vi "Destroy.vi"(0 "reference in":refnum<class "GSwFormDSP.lvclass">, 5 "error in (no error)":errorcluster) -> (14 "reference out":refnum<class "GSwFormDSP.lvclass">, 19 "error out":errorcluster)   [LabVIEW 2022 SP3, in "GSwFormDSP.lvclass"]
doc: "Destructor."
uses:
  GSwFormDSP.lvclass
  Generic Utilities_class/Generic Utilities.lvclass
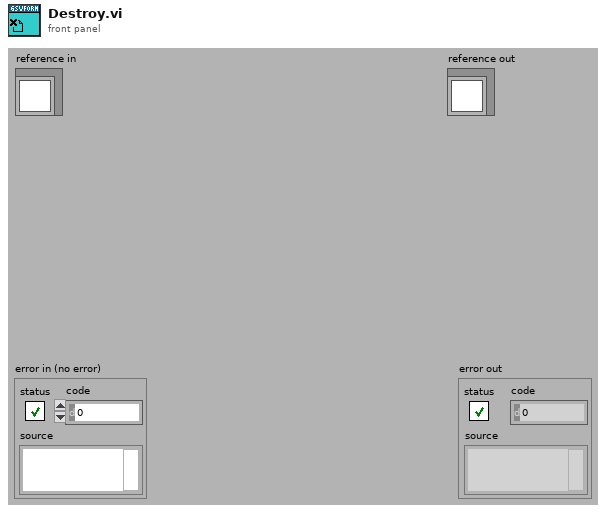
[diagram p1: front panel]
types:
  T1 = typedef "GSwFormDSP.lvclass/ObjectAttributes.ctl" = cluster{"Wform Ref":refnum<data-value>, "Nb Signals":i32, "Spectral Function Parameters":T2, "FFT":waveform(cdb)[], "Nb FFT":i32, "Nb Averages":i32[], "Reference Indexes":i32[], "Response Indexes":i32[], "Coherence":waveform(dbl)[], "TDF Parameters":T4, "DAQ":cluster{"Duration (sec)":dbl, "Buffer Size (Samples)":i32, "Offset (Samples)":i32}, "Filter Impulse Response (TDF)":waveform(dbl), "Sound Playback":T5}
  T2 = typedef "GSwFormDSP.lvclass/Spectral Parameters.ctl" = cluster{"Frequency resolution (Hz)":dbl, "Overlap":dbl, "Window":T3}
  T3 = typedef "NI_AALPro.lvlib/windowTd.ctl" = u32
  T4 = typedef "GSwFormDSP.lvclass/TDF Parameters.ctl" = cluster{"Filter":enum32{"Lowpass", "Highpass", "Bandpass", "Bandstop"}, "Type:":enum16{"Butterworth", "Chebyshev", "Inv Chebyshev", "Elliptic", "Bessel"}, "LP cutoff freq":dbl, "HP cutoff freq":dbl, "Order":i32, "passband ripple (dB)":dbl, "stopband attenuation (dB)":dbl, "Phaseless Filter":bool, "Include Fade IN and OUT":bool}
  T5 = typedef "GSwFormDSP.lvclass/Sound Playback.ctl" = cluster{"Timer start (ms)":u32, "task ID":T6, "Cursor Init Location (s)":dbl, "SC Volume":dbl}
  T6 = typedef "Sound Output Task ID.ctl" = u32
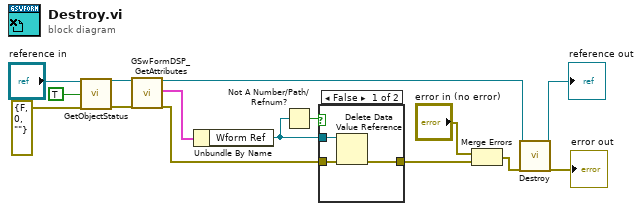
[diagram p0: block diagram]
diagram:
  n1 = call-dynamic "GetObjectStatus.vi"("reference in"="reference in", "simple info (F)"=TRUE ("simple info"), "error in (no error)"=errorcluster {"status"=FALSE, "code"=0, "source"=""}) -> ("reference out"=w9:refnum<class "GSwFormDSP.lvclass">, "error out"=w10:errorcluster)  [unwired: 5 in, 10 out]
  n2 = call "GSwFormDSP_GetAttributes.vi"("reference in"=w9, "error in (no error)"=w10) -> ("reference out"=w8:refnum<class "GSwFormDSP.lvclass">, "attributes"=w7:T1, "error out"=w4:errorcluster)  [unwired: 14 in, 1 out]
  n3 = Unbundle By Name(w7) -> ("Wform Ref"=w2:refnum<data-value>)
  n4 = Not A Number/Path/Refnum?(number/path/refnum=w2) -> (NaN/Path/Refnum?=w1:bool)
  n5 = case shown="False" w1 {
    tunnel: w4 -> [w18 w19]
    tunnel: [w17 w19] -> w3
    tunnel: w2 -> [w16 _]
    frame False {
      n6 = Delete Data Value Reference(data value reference=w16, error in=w18) -> (error out=w17:errorcluster)  [unwired: 1 out]
    }
    frame True {
    }
  }
  n7 = Merge Errors("error in (no error)", w3) -> (w14:errorcluster)
  n8 = call-parent "Destroy.vi"("reference in"=w8, "error in (no error)"=w14) -> ("reference out"=→"reference out":refnum<class "GSwFormDSP.lvclass">, "error out"=→"error out":errorcluster)  [unwired: 16 in]
